vi "Disabled.vi"(7 "Robot Mode":T2, 10 "Match Info":T1={"Autonomous Elapsed Seconds"=0.0, "TeleOp Elapsed Seconds"=0.0, "Disabled Elapsed Seconds"=0.0, "Visited Autonomous"=FALSE, "Visited TeleOp"=FALSE, "Visited Disabled"=FALSE, "Autonomous Settings"={"Autonomous Style"=enum."Independent", "VI Refnum"=refnum}}, 11 "Call Context":T3) -> ()   [LabVIEW 2015]
doc: "This VI is called each time a disabled packet is received from the DS. It is often used to prepare for the next robot mode, to calibrate sensors, etc."
uses:
  <vilib>/Rock Robotics/WPI/DriverStation/WPI_DriverStationDerivedRobotMode.ctl
  <vilib>/Rock Robotics/WPI/DriverStation/WPI_DriverStationRobotMode2.ctl
  <vilib>/Rock Robotics/WPI/DriverStation/WPI_DriverStationMatch Info.ctl
  Common Code/Shooter Commands.ctl
  Common Code/Intake Commands.ctl
  Common Code/Change Detect.vi
  Common Code/Change Detect Boolean.vi
  <vilib>/Rock Robotics/WPI/Utilities/WPI_GetSetVariantRefNum.vi
  Robot Global Data.vi
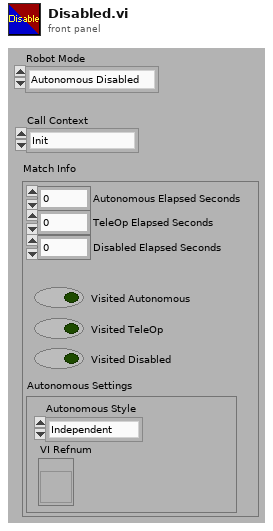
[diagram p1: front panel]
types:
  T1 = typedef "WPI_DriverStationMatch Info.ctl" = cluster{"Autonomous Elapsed Seconds":dbl, "TeleOp Elapsed Seconds":dbl, "Disabled Elapsed Seconds":dbl, "Visited Autonomous":bool, "Visited TeleOp":bool, "Visited Disabled":bool, "Autonomous Settings":cluster{"Autonomous Style":enum16{"Iterative", "Independent"}, "VI Refnum":refnum<vi>}}
  T2 = typedef "WPI_DriverStationRobotMode2.ctl" = enum16{"Autonomous Disabled", "Autonomous Enabled", "Teleop Disabled", "Teleop Enabled", "Disconnected", "Finish", "Test Disabled", "Test Enabled", "Emergency Stopped"}
  T3 = typedef "WPI_DriverStationDerivedRobotMode.ctl" = enum16{"Init", "Execute", "Stop"}
  T4 = enum16{"0", "1", "2", "3", "4", "5", "6", "7", "8", "9", "A", "B", "C", "D", "E", "F", "G", "H", "I", "J", "K", "L", "M", "N", "O", "P", "Q", "R", "S", "T", "U", "V", "W", "X", "Y", "Z", "F1", "F2", "F3", "F4", "F5", "F6", "F7", "F8", "F9", "F10", "F11", "F12", "F13", "F14", "F15", "ADD", "BACK", "BACKSLASH", "CAPITAL", "COMMA", "DECIMAL", "DELETE", "DIVIDE", "DOWN", "END", "EQUALS", "ESCAPE", "GRAVE (`)", "HOME", "INSERT", "LBRACKET", "LCONTROL", "LEFT", "L ALT", "LSHIFT", "LWIN", "MINUS", "MULTIPLY", "NEXT", "NUMLOCK", "NUMPAD_0", "NUMPAD_1", "NUMPAD_2", "NUMPAD_3", "NUMPAD_4", "NUMPAD_5", "NUMPAD_6", "NUMPAD_7", "NUMPAD_8", "NUMPAD_9", "PAUSE", "PERIOD", "PRIOR (PG UP)", "RBRACKET", "RCONTROL", "RETURN", "RIGHT", "R ALT", "RSHIFT", "RWIN", "SCROLL", "SEMICOLON", "SLASH", "SPACE", "SUBTRACT", "TAB", "UP", "ENTER (num pad)", "' (quote)"}
  T5 = typedef "Intake Commands.ctl" = enum16{"Unload", "Load", "Pull up", "Drop low", "Idle", "Lift Half"}
  T6 = typedef "Shooter Commands.ctl" = enum16{"Idle", "Prime Shooter", "Shoot"}
  T7 = typedef "WPI_JoystickDevRef.ctl" = cluster{"Device":T8}
  T8 = typedef "WPI_JoystickDeviceEnum.ctl" = enum16{"USB 0", "USB 1", "USB 2", "USB 3", "USB 4", "USB 5"}
  T9 = typedef "Intake Mode.ctl" = enum16{"Safe", "Auto", "Manual"}
  T10 = typedef "Intake Commands Cluster.ctl" = cluster{"Intake Commands":T5, "Intake Mode":T9}
  T11 = typedef "Climb Command Cluster.ctl" = cluster{"Climb Mode":T12, "Hold?":bool, "Manual State":T13}
  T12 = typedef "Climb Mode.ctl" = enum16{"Auto", "Manual"}
  T13 = typedef "Climb Manual State.ctl" = cluster{"Release":bool, " PTO Engage":bool}
  T14 = typedef "D-Pad.ctl" = cluster{"Top":bool, "Bottom":bool, "None":bool, "Right":bool, "Left":bool}
  T15 = typedef "Button Cluster.ctl" = cluster{"Buttons[0]":bool, "Buttons[1]":bool, "Buttons[2]":bool, "Buttons[3]":bool, "Buttons[4]":bool, "Buttons[5]":bool, "Buttons[6]":bool, "Buttons[7]":bool, "Buttons[8]":bool, "Buttons[9]":bool}
  T16 = typedef "Shooter Command Cluster.ctl" = cluster{"Command":T6, "Mode":T17, "Shot Type":T18, "Override Trigger IR":bool, "Override Angle?":bool}
  T17 = typedef "Shoot Modes Enum.ctl" = enum16{"Manual", "Safe", "Auto"}
  T18 = typedef "Shot Type.ctl" = enum16{"Batter Shot", "Corner Shot", "Curve Shot", "Vision Shot", "Deep Middle Shot"}
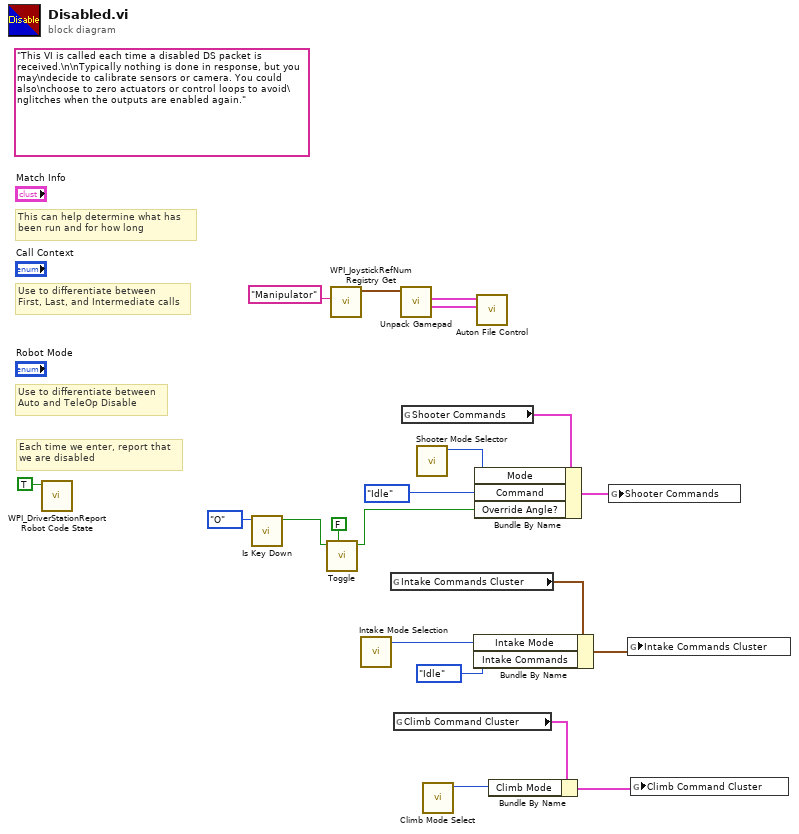
[diagram p0: block diagram]
diagram:
  (unwired) "This VI is called each time a disabled DS packet is received.\n\nTypically nothing is done in response, but you may\ndecide to calibrate sensors or camera. You could also\nchoose to zero actuators or control loops to avoid\nglitches when the outputs are enabled again."
  # "Each time we enter, report that\nwe are disabled"
  # "Use to differentiate between\nFirst, Last, and Intermediate calls"
  # "This can help determine what has\nbeen run and for how long"
  # "Use to differentiate between\nAuto and TeleOp Disable"
  n1 = call <vilib>:"WPI_DriverStationReport Robot Code State.vi"("Disabled"=TRUE ("Autonomous")) -> ()  [unwired: 10 in, 1 out]
  n2 = call "Is Key Down.vi"("Key"=T4."O") -> ("Key Down?"=w4:bool)  [unwired: 10 in]
  n3 = call "Toggle.vi"("Initial Value"=FALSE, "In"=w4) -> ("Toggled"=w1:bool)  [unwired: 9 in]
  n4 = call <vilib>:"WPI_JoystickRefNum Registry Get.vi"("refnum name"="Manipulator") -> ("JoystickDevRef"=w18:T7)  [unwired: 1 in, 9 out]
  n5 = call "Intake Mode Selection.vi"() -> ("Mode"=w8:T9)  [unwired: 11 in]
  n6 = global read "Robot Global Data.vi" "Intake Commands Cluster"() -> (w10:T10)
  n7 = global read "Robot Global Data.vi" "Climb Command Cluster"() -> (w7:T11)
  n8 = call "Unpack Gamepad.vi"("JoystickDevRef"=w18) -> ("D-Pad"=w16:T14, "Button Cluster"=w17:T15)  [unwired: 8 in, 1 out]
  n9 = global read "Robot Global Data.vi" "Shooter Commands"() -> (w15:T16)
  n10 = call "Shooter Mode Selector.vi"() -> ("Mode"=w14:T17)  [unwired: 11 in]
  n11 = call "Climb Mode Select.vi"() -> ("Mode"=w5:T12)  [unwired: 11 in]
  n12 = Bundle By Name(cluster=w10, "Intake Mode"=w8, "Intake Commands"=Intake_Commands."Idle") -> (w11:T10)
  n13 = Bundle By Name(cluster=w15, "Mode"=w14, "Command"=Shooter_Commands."Idle", "Override Angle?"=w1) -> (w12:T16)
  n14 = call "Auton File Control.vi"("Manip D-Pad"=w16, "Manip Button"=w17) -> ()  [unwired: 10 in]
  n15 = Bundle By Name(cluster=w7, "Climb Mode"=w5) -> (w6:T11)
  n16 = global write "Robot Global Data.vi" "Shooter Commands"(w12) -> ()
  n17 = global write "Robot Global Data.vi" "Intake Commands Cluster"(w11) -> ()
  n18 = global write "Robot Global Data.vi" "Climb Command Cluster"(w6) -> ()
